vi "CSP_SortEigenvalues.vi"(10 "Eigenvectors":T1, 11 "Eigenvalues":cdb[](array[numeric]) format="%.2f") -> (2 "Eigenvectors Sorted":T1, 3 "Eigenvalues Sorted":dbl[](array[numeric]))   [LabVIEW 2016, in "Spatial Pattern Filter.lvlib"]
uses:
  <vilib>/Analysis/Matrix/Datatypes/ComplexMatrix.ctl
  <vilib>/Analysis/Matrix/Numeric/Conversions/Array To Matrix - CA2.vi
  Spatial Pattern Filter.lvlib
  <vilib>/Analysis/Matrix/NI_Matrix.lvlib
panel:
  # "This VI is a part of BCI Design library, http://www.ru-bci.org \nCopyright © 2020, Sotnikov Peter, All rights reserved. License: CC BY-NC 4.0"
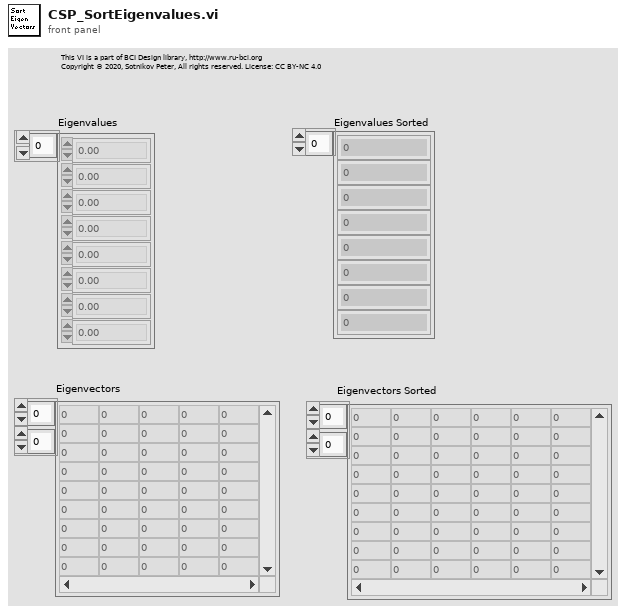
[diagram p1: front panel]
types:
  T1 = typedef "NI_Matrix.lvlib/ComplexMatrix.ctl" = cdb[][]
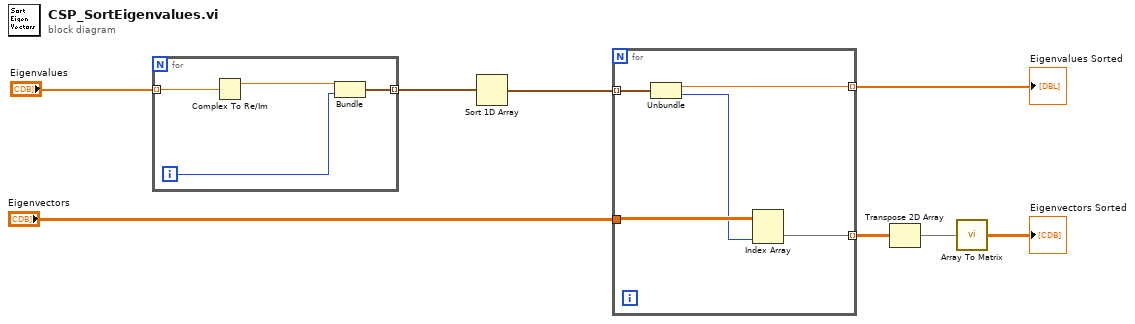
[diagram p0: block diagram]
diagram:
  n1 = for {
    tunnel: "Eigenvalues" -> [w10] mode=indexing
    tunnel: [w11] -> w7 mode=indexing
    i -> [w12]
    n2 = Complex To Re/Im(x + iy=w10) -> (x=w9:dbl)  [unwired: 1 out]
    n3 = Bundle(w9, w12) -> (w11:cluster{dbl, i32})  [unwired: 1 in]
  }
  n4 = Sort 1D Array(array=w7) -> (sorted array=w6:cluster{dbl, i32}[])
  n5 = for {
    tunnel: w6 -> [w17] mode=indexing
    tunnel: "Eigenvectors" -> [w16]
    tunnel: [w15] -> w3 mode=indexing
    tunnel: [w14] -> w2 mode=indexing
    n6 = Unbundle(w17) -> (w15:dbl, w13:i32)
    n7 = Index Array(array=w16, index (col)=w13) -> (element=w14:cdb[])  [unwired: 1 in]
  }
  "Eigenvalues Sorted" <- w3
  n8 = Transpose 2D Array(2D array=w2) -> (transposed array=w1:cdb[][])
  n9 = call-poly <vilib>:"Array To Matrix.vi"("Complex 2D Array"=w1) -> ("Complex Matrix"=→"Eigenvectors Sorted":T1)
